vi "Get Active Worksheet Name.vi"(0 "Report Ref In":T1, 1 "error in (no error)":errorcluster) -> (2 "Report Ref Out":T1, 3 "Worksheet Name":string, 4 "error out":errorcluster)   [LabVIEW 2013, in "XCel Report Engine.lvlib"]
doc: "Returns the name of the worksheet currently selected in the open report session.\n\nThe active worksheet determines which worksheet is used by subsequent cell, range, image, and formatting operations.\n\nThis VI does not modify the workbook or change the active worksheet."
uses:
  XCel Report Engine.lvlib
  C:/Users/m.santucci/Documents/ChatGPT/LV_REPORT_ENGINE/LV/DotNet/XCelReportEngine.dll
  LV/DotNet/XCelReportEngine.dll
  Controls/Report Ref.ctl
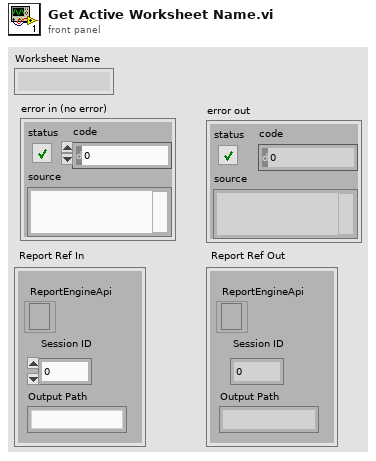
[diagram p1: front panel]
types:
  T1 = typedef "XCel Report Engine.lvlib/Report Ref.ctl" = cluster{"Session ID":i32, "Output Path":string, "ReportEngineApi":refnum<k24>}
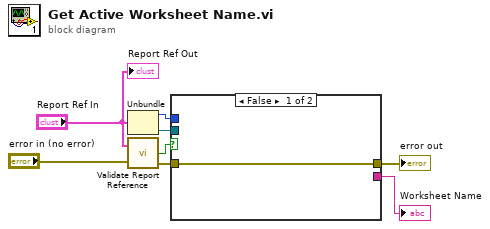
[diagram p0: block diagram]
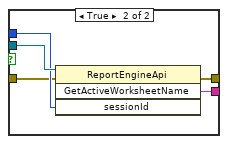
[diagram p2: hidden frame]
diagram:
  n1 = Unbundle("Report Ref In") -> ("Session ID"=w7:i32, "ReportEngineApi"=w8:refnum<k24>)  [unwired: 1 out]
  n2 = call "Validate Report Reference.vi"("Report Ref In"="Report Ref In", "error in (no error)"="error in (no error)") -> ("Valid"=w1:bool, "error out"=w3:errorcluster)  [unwired: 1 out]
  n3 = case shown="False" w1 {
    tunnel: w8 -> [_ w14]
    tunnel: w7 -> [_ w13]
    tunnel: [w9 w12] -> w6
    tunnel: [_ w11] -> w5
    tunnel: w3 -> [w9 w10]
    frame False {
    }
    frame True {
      n4 = invoke class="ReportEngineApi" method="GetActiveWorksheetName"(reference=w14, error in=w10, "sessionId"=w13) -> (error out=w12:errorcluster, "GetActiveWorksheetName"=w11:string)  [unwired: 1 in, 2 out]
    }
  }
  "error out" <- w6
  "Worksheet Name" <- w5
  "Report Ref Out" <- "Report Ref In"
